vi "SetTypeMap.vi"(8 "error in (no error)":errorcluster, 10 "TypeMap in":refnum<class "TypeMap.lvclass">, 11 "object in":refnum<class>) -> (0 "error out":errorcluster, 2 "replaced?":bool, 3 "object out":refnum<class>)   [LabVIEW 2020, in "ORM_API.lvlib"]
uses:
  ORM_API.lvlib
  <vilib>/Viviota/shared/ORM.lvlibp/ORM/TypeMap/TypeMap.lvclass
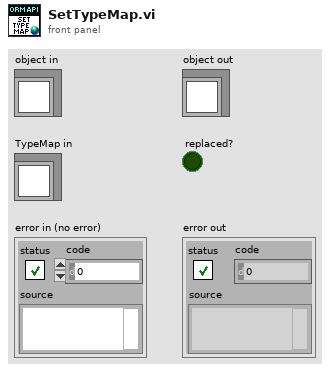
[diagram p1: front panel]
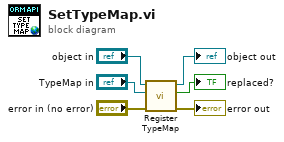
[diagram p0: block diagram]
diagram:
  n1 = call <vilib>:"Register TypeMap.vi"("error in (no error)"="error in (no error)", "TypeMap in"="TypeMap in", "object in"="object in") -> ("error out"=→"error out":errorcluster, "replaced?"=→"replaced?":bool, "object out"=→"object out":refnum<class>)  [unwired: 6 in]
